vi "Is x divisible by y.vi"(8 "error in (no error)":errorcluster, 10 "y":i32, 11 "x":i32) -> (0 "error out":errorcluster, 2 "floor (x/y)":i32, 3 "T = x is divisible by y":bool)   [LabVIEW 2021, in "Numeric Utilities.lvlib"]
uses:
  Numeric Utilities.lvlib
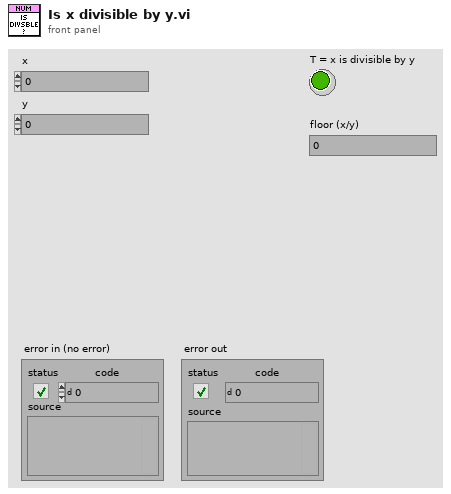
[diagram p1: front panel]
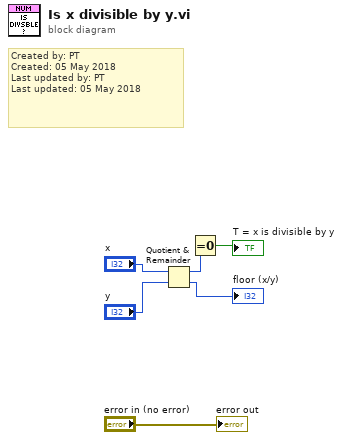
[diagram p0: block diagram]
diagram:
  # "Created by: PT\nCreated: 05 May 2018\nLast updated by: PT\nLast updated: 05 May 2018"
  n1 = Quotient & Remainder(x="x", y="y") -> (x-y*floor(x/y)=w2:i32, floor(x/y)=→"floor (x/y)":i32)
  n2 = Equal To 0?(x=w2) -> (x = 0?=→"T = x is divisible by y":bool)
  "error out" <- "error in (no error)"
